vi "Latching_Boolean_Array.vi"() -> ()   [LabVIEW 2018]
panel:
  out "Button Pressed":i32
  in  "stop":bool
  in  "Array":bool[](array[boolean])=[FALSE, FALSE, FALSE, FALSE, FALSE, FALSE, FALSE, FALSE]
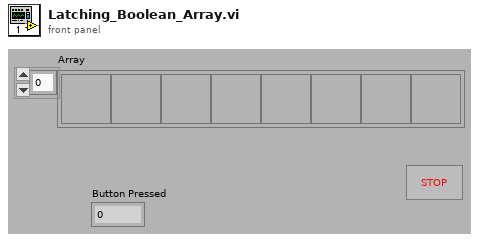
[diagram p1: front panel]
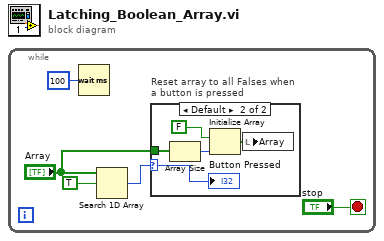
[diagram p0: block diagram]
diagram:
  n1 = while {
    stop <- "stop" stop-if-true
    n2 = Wait (ms)(milliseconds to wait=u32 100) -> ()  [unwired: 1 out]
    n3 = Search 1D Array(1D array="Array", element=TRUE) -> (index of element=w3:i32)  [unwired: 1 in]
    n4 = case "Reset array to all Falses when\na button is pressed" shown="Default" w3 {
      selector: w3 -> [_ w6]
      tunnel: "Array" -> [_ w10]
      frame -1 {
        # "Do not write to array\nwhen idle to avoid a\nrace condition"
      }
      frame Default {
        n5 = Array Size(array=w10) -> (size(s)=w9:i32)
        n6 = Initialize Array(FALSE ("element"), w9) -> (w7:bool[])
        n7 = local write "Array"(w7) -> ()
        "Button Pressed" <- w6
      }
    }
  }
